vi "Check for Valid Device.vi"(8 "error in (no error)":errorcluster, 11 "device in":refnum<class "NI_Robotics_Starter Kit Direct IO_FPGA.lvclass">) -> (0 "error out":errorcluster, 2 "valid?":bool, 3 "device out":refnum<class "NI_Robotics_Starter Kit Direct IO_FPGA.lvclass">)   [LabVIEW 2017, in "NI_Robotics_Starter Kit Direct IO_FPGA.lvclass"]
uses:
  <vilib>/robotics/Starter Kit/FPGA Direct IO/NI_Robotics_Starter Kit Direct IO_FPGA.lvclass
  <vilib>/robotics/Starter Kit/FPGA Direct IO/NI_Robotics_Starter Kit Direct IO_FPGA.lvclass/NI_Robotics_Starter Kit Direct IO_FPGA.ctl
  <vilib>/robotics/Starter Kit/Direct IO/NI_Robotics_Starter Kit Direct IO.lvclass
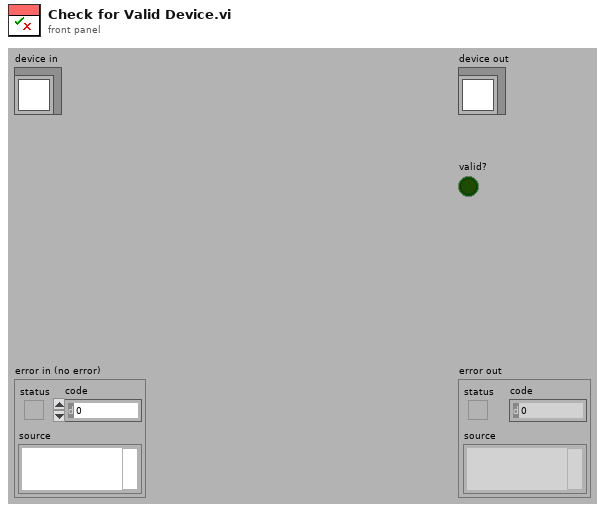
[diagram p1: front panel]
types:
  T1 = typedef "NI_Robotics_Starter Kit Direct IO_FPGA.lvclass/Direct IO FPGA Ref.ctl" = refnum<k20>
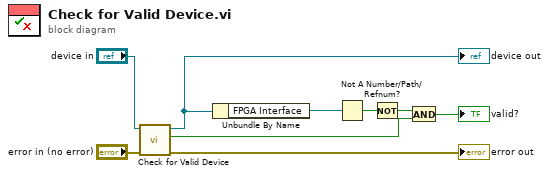
[diagram p0: block diagram]
diagram:
  n1 = call-parent "Check for Valid Device.vi"("error in (no error)"="error in (no error)", "device in"="device in") -> ("error out"=→"error out":errorcluster, "valid?"=w2:bool, "device out"=w6:refnum<class "NI_Robotics_Starter Kit Direct IO_FPGA.lvclass">)  [unwired: 7 in]
  "device out" <- w6
  n2 = Unbundle By Name(w6) -> ("FPGA Interface"=w5:T1)
  n3 = Not A Number/Path/Refnum?(number/path/refnum=w5) -> (NaN/Path/Refnum?=w4:bool)
  n4 = Not(x=w4) -> (.not. x?=w3:bool)
  n5 = And(x=w3, y=w2) -> (x .and. y?=→"valid?":bool)
